vi "ReadM1PositionPID.vi"() -> ()   [LabVIEW 2015]
uses:
  <instrlib>/Ion Motion Roboclaw/Ion Motion Roboclaw.lvlib
panel:
  in  "Address":u8
  out "Deadzone":u32
  out "MinPos":u32
  out "MaxPos":u32
  out "KiMax":u32
  out "Valid":bool
  out "Kd":u32
  out "Ki":u32
  out "Kp":u32
  out "error out":errorcluster
  in  "COM port":refnum<visa-resource-name>
  in  "baud rate (38400)":u32
  in  "error in (no error)":errorcluster
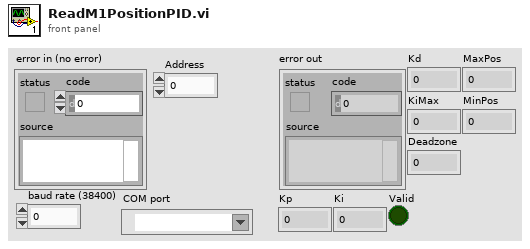
[diagram p1: front panel]
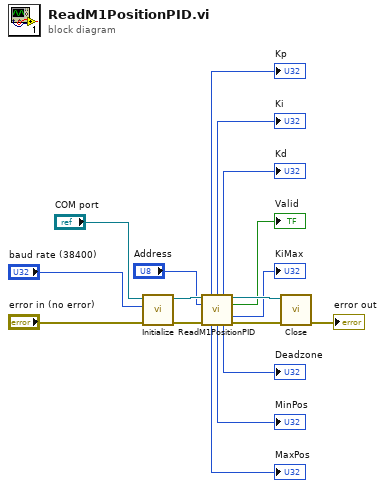
[diagram p0: block diagram]
diagram:
  n1 = call <instrlib>:"Initialize.vi"("error in (no error)"="error in (no error)", "baud rate (38400)"="baud rate (38400)", "COM port"="COM port") -> ("error out"=w16:errorcluster, "VISA resource name out"=w17:refnum<visa-resource-name>)  [unwired: 7 in]
  n2 = call <instrlib>:"ReadM1PositionPID.vi"("VISA Refnum in"=w17, "Address"="Address", "error in (no error)"=w16) -> ("Kp"=→"Kp":u32, "Ki"=→"Ki":u32, "Kd"=→"Kd":u32, "VISA Refnum out"=w15:refnum<visa-resource-name>, "Valid"=→"Valid":bool, "KiMax"=→"KiMax":u32, "MaxPos"=→"MaxPos":u32, "MinPos"=→"MinPos":u32, "Deadzone"=→"Deadzone":u32, "error out"=w14:errorcluster)  [unwired: 3 in]
  n3 = call <instrlib>:"Close.vi"("error in (no error)"=w14, "VISA resource name"=w15) -> ("error out"=→"error out":errorcluster)  [unwired: 9 in]
